vi "Do This.vi"(8 "error in (no error)":errorcluster, 10 "Status Events":refnum<class "Status Events.lvclass">, 11 "VIPC Apply in":refnum<class "VIPC Apply.lvclass">) -> (0 "error out":errorcluster, 3 "VIPC Apply out":refnum<class "VIPC Apply.lvclass">)   [LabVIEW 2014, in "VIPC Apply.lvclass"]
uses:
  VIPC Apply.lvclass
  Classes/Status Events/Status Events.lvclass
  VIPC Apply.lvclass/VIPC Apply.ctl
  <vilib>/Utility/error.llb/DialogType.ctl
  Classes/Job/Job.lvclass/Job.ctl
  Classes/Job/Job.lvclass
  <vilib>/JKI/VIPM API/VIPM API_vipm_api.lvlib
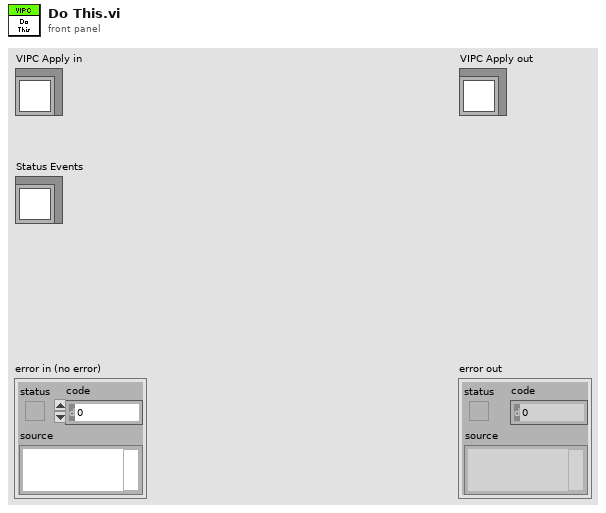
[diagram p1: front panel]
types:
  T1 = typedef "DialogType.ctl" = u16
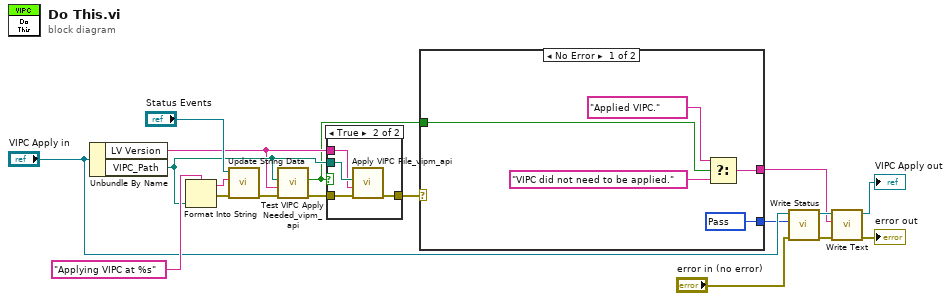
[diagram p0: block diagram]
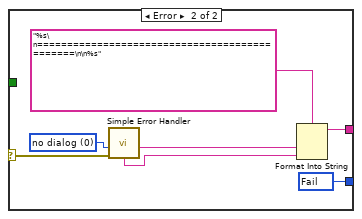
[diagram p3: hidden frame]
diagram:
  n1 = Unbundle By Name("VIPC Apply in") -> ("LV Version"=w2:string, "VIPC_Path"=w3:path)
  n2 = Format Into String(format string="Applying VIPC at %s", w3) -> (resulting string=w17:string, error out=w9:errorcluster)  [unwired: 2 in]
  n3 = call "Update String Data.vi"("error in (no error)"=w9, "String Data"=w17, "Status Updater in"="Status Events") -> ("error out"=w4:errorcluster)  [unwired: 7 in, 1 out]
  n4 = call <vilib>:"Test VIPC Apply Needed_vipm_api.vi"("error in (no error)"=w4, "LabVIEW Version (use vipc version)"=w2, "VIPC File Path"=w3) -> ("error out"=w5:errorcluster, "Need to Apply?"=w1:bool)  [unwired: 7 in]
  n5 = case shown="True" w1 {
    tunnel: w5 -> [w19 w23]
    tunnel: [w19 w22] -> w8
    tunnel: w3 -> [_ w21]
    tunnel: w2 -> [_ w20]
    frame False {
    }
    frame True {
      n6 = call <vilib>:"Apply VIPC File_vipm_api.vi"("error in (no error)"=w23, "LabVIEW Version"=w20, "VIPC File"=w21) -> ("error out"=w22:errorcluster)  [unwired: 8 in]
    }
  }
  n7 = case shown="No Error" w8 {
    selector: w8 -> [_ w34]
    tunnel: [w28 w35] -> w11
    tunnel: [w24 w29] -> w12
    tunnel: w1 -> [w27 _]
    frame No Error {
      w28 = u16 200 items=["Abort"=503, "Fail"=500, "Pass"=200] ("Status")
      n8 = Select(t="Applied VIPC." ("Text"), s=w27, f="VIPC did not need to be applied.") -> (s? t:f=w24:string)
    }
    frame Error {
      w33 = T1 0 items=["no dialog", "OK message", "continue or stop message", "OK message + warnings", "continue/stop + warnings"] ("type of dialog (OK msg:1)")
      w35 = u16 500 items=["Abort"=503, "Fail"=500, "Pass"=200] ("Status")
      n9 = call <vilib>:"Simple Error Handler.vi"("type of dialog (OK msg:1)"=w33, "error in (no error)"=w34) -> ("source out"=w31:string, "message"=w30:string)  [unwired: 3 in, 3 out]
      n10 = Format Into String(format string="%s\n==============================================\n\n%s", w31, w30) -> (resulting string=w29:string)  [unwired: 2 in, 1 out]
    }
  }
  n11 = call "Write Status.vi"("error in (no error)"="error in (no error)", "Status"=w11, "Job in"="VIPC Apply in") -> ("error out"=w13:errorcluster, "Job out"=w14:refnum<class "VIPC Apply.lvclass">)  [unwired: 7 in]
  n12 = call "Write Text.vi"("error in (no error)"=w13, "Text"=w12, "Job in"=w14) -> ("error out"=→"error out":errorcluster, "Job out"=→"VIPC Apply out":refnum<class "VIPC Apply.lvclass">)  [unwired: 7 in]
